vi "MB MFC Setpoint.vi"(7 "Action":T1, 8 "error in (no error)":errorcluster, 9 "Setpoint":sgl, 11 "TCP Ref":refnum<k5>) -> (0 "error out":errorcluster, 1 "Setpoint":sgl, 3 "dup TCP Ref":refnum<k5>)   [LabVIEW 2015]
doc: "This VI reads or writes a setpoint to an MKS Modbus MFC. This VI provides no checking that the setpoint was accepted by the device."
uses:
  Type Definitions/Modbus Action.ctl
  subVIs/MKS/EtherNet.lib/Modbus/mb Ethernet.llb/MB Modbus Command.ctl
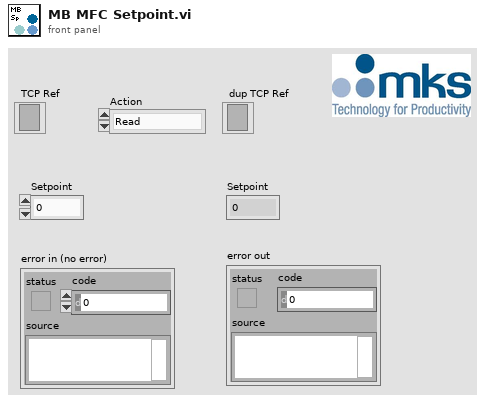
[diagram p1: front panel]
types:
  T1 = typedef "Modbus Action.ctl" = enum16{"Read", "Write"}
  T2 = typedef "MB Modbus Command.ctl" = cluster{"Function Code":u8, "Starting Address":u16, "Quantity":u16, "Data":u16[], "Discrete":bool[]}
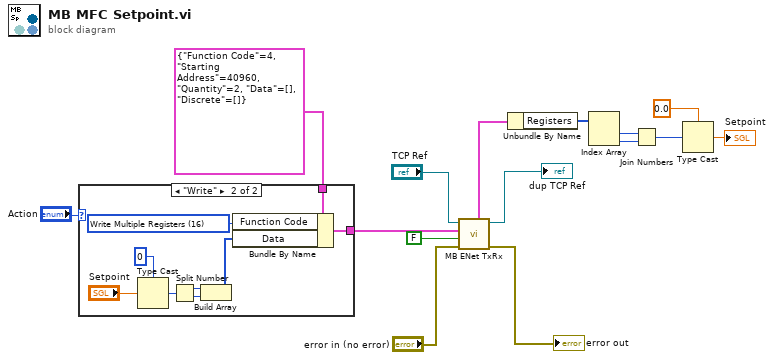
[diagram p0: block diagram]
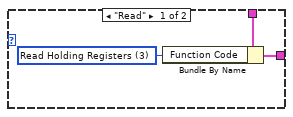
[diagram p2: hidden frame]
diagram:
  n1 = case shown="\"Write\"" "Action" {
    tunnel: T2 {"Function Code"=4, "Starting Address"=40960, "Quantity"=2, "Data"=[], "Discrete"=[]} ("Modbus Command") -> [w18 w27]
    tunnel: [w17 w26] -> w1
    frame "Read" {
      w16 = u8 3 items=["Read Coils"=1, "Read Discrete Inputs"=2, "Read Holding Registers"=3, "Read Input Registers"=4, "Write Single Coil"=5, "Write Single Register"=6, "Read Exception Status"=7, "Write Multiple Coils"=15, "Write Multiple Registers"=16, "Read Device Id"=43] ("Function Code")
      n2 = Bundle By Name(cluster=w18, "Function Code"=w16) -> (w17:T2)
    }
    frame "Write" {
      w25 = u8 16 items=["Read Coils"=1, "Read Discrete Inputs"=2, "Read Holding Registers"=3, "Read Input Registers"=4, "Write Single Coil"=5, "Write Single Register"=6, "Read Exception Status"=7, "Write Multiple Coils"=15, "Write Multiple Registers"=16, "Read Device Id"=43] ("Function Code")
      n3 = Type Cast(type=u32 0 ("element"), x="Setpoint") -> (*(type *) &x=w22:u32)
      n4 = Split Number(x=w22) -> (hi(x)=w21:u16, lo(x)=w20:u16)
      n5 = Build Array(w21, w20) -> (w19:u16[])
      n6 = Bundle By Name(cluster=w27, "Function Code"=w25, "Data"=w19) -> (w26:T2)
    }
  }
  n7 = call "MB ENet TxRx.vi"("error in (no error)"="error in (no error)", "Use MODBUS Data Unit?"=FALSE, "Modbus Command"=w1, "TCP Ref:ValBlock"="TCP Ref") -> ("error out"=→"error out":errorcluster, "dup TCP Ref:ValBlock"=→"dup TCP Ref":refnum<k5>, "Registers"=w14:cluster{"Registers":u16[], "Discrete":bool[]})  [unwired: 3 in, 2 out]
  n8 = Unbundle By Name(w14) -> ("Registers"=w13:u16[])
  n9 = Index Array(array=w13) -> (element #1=w12:u16, element #2=w11:u16)  [unwired: 2 in]
  n10 = Join Numbers(hi=w12, lo=w11) -> ((hi.lo)=w10:u32)
  n11 = Type Cast(type=sgl 0.0 ("element"), x=w10) -> (*(type *) &x=→"Setpoint":sgl)
